vi "PS2521G_ONvi.vi"(7 "GPIB Bus":i32 min=0 max=5, 8 "error in":errorcluster, 11 "GPIB Address":i16=8 max=31) -> (0 "error out":errorcluster)   [LabVIEW 2023]
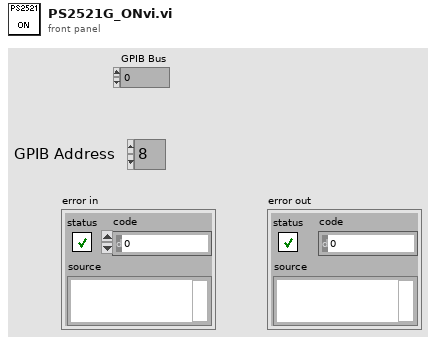
[diagram p1: front panel]
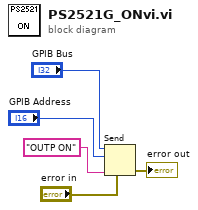
[diagram p0: block diagram]
diagram:
  n1 = Send(0:"GPIB Bus", 2:"GPIB Address", 4:"error in", 5:"OUTP ON" ("data string")) -> (8:→"error out":errorcluster)  [unwired: 1 in, 2 out]
